vi "Write Data in CVT.vi"(8 "error in (no error)":errorcluster, 11 "Read Buffer":string) -> (0 "error out":errorcluster, 3 "Channel Data":string[](array[string]))   [LabVIEW 2016, in "Serial Hardware.lvlib"]
uses:
  Serial Hardware.lvlib
  <vilib>/NI/Current Value Table/Type Defs/Group Data.ctl
  <vilib>/NI/Current Value Table/DataTypes/Array of Double_Read.vi
  <vilib>/NI/Current Value Table/Type to Enum.vi
  <vilib>/NI/Current Value Table/DataTypes/Array of Double_Type To Enum.vi
  <vilib>/NI/Current Value Table/FGVs/CVT Globals.vi
  <vilib>/NI/Current Value Table/FGVs/Tag Memory.vi
  <vilib>/NI/Current Value Table/Memory Block.vi
  <vilib>/NI/Current Value Table/DataTypes/Array of Double_Memory Block.vi
  <vilib>/NI/Current Value Table/Current Value Table.lvlib
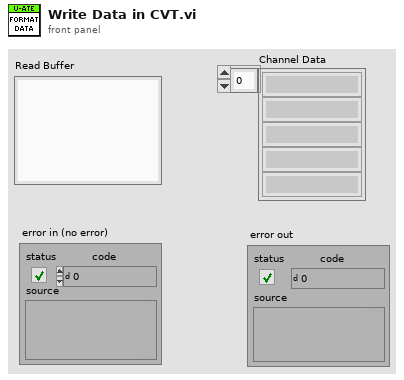
[diagram p1: front panel]
types:
  T1 = typedef "Current Value Table.lvlib/Group Data.ctl" = cluster{"Double":dbl[], "Single":sgl[], "I64":i64[], "I32":i32[], "I16":i16[], "I8":i8[], "U64":u64[], "U32":u32[], "U16":u16[], "U8":u8[], "String":string[], "Boolean":bool[], "Array of U8":cluster{"U8 Array":u8[]}[], "Array of U16":cluster{"U16 Array":u16[]}[], "Array of U32":cluster{"U32 Array":u32[]}[], "Array of U64":cluster{"U64 Array":u64[]}[], "Array of I64":cluster{"I64 Array":i64[]}[], "Array of I32":cluster{"I32 Array":i32[]}[], "Array of I16":cluster{"I16 Array":i16[]}[], "Array of I8":cluster{"I8 Array":i8[]}[], "Array of Double":cluster{"DBL Array":dbl[]}[], "Array of Single":cluster{"SGL Array":sgl[]}[], "Array of Boolean":cluster{"Boolean Array":bool[]}[], "Array of String":cluster{"String Array":string[]}[]}
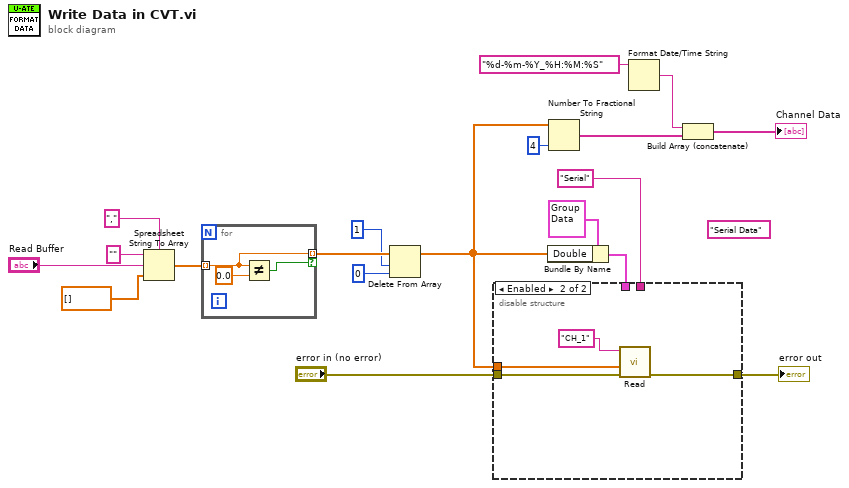
[diagram p0: block diagram]
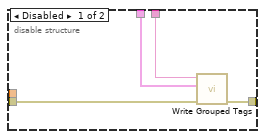
[diagram p2: hidden frame]
diagram:
  (unwired) "Serial Data" ("Group")
  n1 = Spreadsheet String To Array(delimiter (Tab)=",", format string="", spreadsheet string="Read Buffer", array type (2D Dbl)=dbl[] []) -> (array=w15:dbl[])
  n2 = for {
    tunnel: w15 -> [w21] mode=indexing
    tunnel: [w21] -> w10 mode=indexing if=w20
    n3 = Not Equal?(x=w21, y=0.0) -> (x != y?=w20:bool)
  }
  n4 = Delete From Array(array=w10, length=1, index=0) -> (array with subset deleted=w2:dbl[])  [unwired: 1 out]
  n5 = Bundle By Name(cluster=T1 {"Double"=[], "Single"=[], "I64"=[], "I32"=[], "I16"=[], "I8"=[], "U64"=[], "U32"=[], "U16"=[], "U8"=[], "String"=[], "Boolean"=[], "Array of U8"=[], "Array of U16"=[], "Array of U32"=[], "Array of U64"=[], "Array of I64"=[], "Array of I32"=[], "Array of I16"=[], "Array of I8"=[], "Array of Double"=[], "Array of Single"=[], "Array of Boolean"=[], "Array of String"=[]} ("Data"), "Double"=w2) -> (w13:T1)
  n6 = disable-structure shown="Enabled" {
    disable-tunnel: "Serial" ("Group") -> [w26 _]
    disable-tunnel: w13 -> [w25 _]
    disable-tunnel: [w24 w27] -> w12
    disable-tunnel: "error in (no error)" -> [w23 w28]
    disable-tunnel: w2 -> [_ w29]
    frame Disabled {
      n7 = call <vilib>:"Write Grouped Tags.vi"("error in (no error)"=w23, "Data"=w25, "Group"=w26) -> ("error out"=w24:errorcluster)  [unwired: 8 in]
    }
    frame Enabled {
      n8 = call-poly <vilib>:"Read.vi"("error in (no error)"=w28, "Default"=w29, "Tag Name"="CH_1") -> ("error out"=w27:errorcluster)  [unwired: 7 in, 1 out]
    }
  }
  "error out" <- w12
  n9 = Number To Fractional String(number=w2, precision (6)=i16 4) -> (F-format string=w8:string[])  [unwired: 2 in]
  n10 = Format Date/Time String(time format string (%c)="%d-%m-%Y_%H:%M:%S") -> (date/time string=w5:string)  [unwired: 2 in]
  n11 = Build Array (concatenate)(w5, w8) -> (→"Channel Data":string[])
